vi "InitAction(poly).vi"   [LabVIEW 2024, in "ActionStack.lvlib" / "Action.lvclass"]
uses:
  Action.lvclass
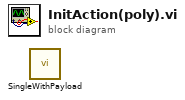
[diagram p0: block diagram]
diagram:
  n1 = call "SingleWithPayload.vi"() -> ()  [unwired: 11 in, 1 out]
